vi "dC(T)_2024.vi"(2 "Temperature (K)":dbl=373.15 format="%.4g") -> (0 "dCa/dT":dbl=-9.989510208451924e-13 format="%#_4g", 1 "d^2Ca/dT^2":dbl=2.3734887970956986e-15 format="%#_4g", 3 "dCw/dT":dbl=1.21722616713758e-08 format="%_4g", 4 "d^2Cw/dT^2":dbl=-3.6083232318005423e-10 format="%_4g", 5 "T*dCa/dT":dbl=-3.7275857342838354e-10 format="%#_4g", 6 "T^2*d^2Ca/dT^2":dbl=3.3048676965102036e-10 format="%#_4g", 8 "T*dCw/dT":dbl=4.54207944267388e-06 format="%#_4g", 9 "T^2*d^2Cw/dT^2":dbl=-5.024262554740888e-05 format="%_4e")   [LabVIEW 2016]
uses:
  2022/SOS_Global_2022.vi
  <vilib>/Analysis/NI_AALPro.lvlib
  <vilib>/gmath/NI_Gmath.lvlib
panel:
  in  "C source ref water":i32(listbox)=1
  in  "C source ref dry air":i32(listbox)=1
  in  "method derivatives":u16(ring)=2 items=["2nd Order Central", "4th Order Central", "Forward", "Backward"]
  in  "interpolation method":i32(ring)=2 items=["nearest", "linear", "spline", "cubic Hermite", "Lagrange"]
  in  "method interpolation":i32(ring)=2 items=["nearest", "linear", "spline", "cubic Hermite", "Lagrange"]
  in  "method derivatives":u16(ring)=2 items=["2nd Order Central", "4th Order Central", "Forward", "Backward"]
  # "m^6/mol^2"
  # "m^6/(mol^2 K)"
  # "m^6/(mol^2 K^2)"
  # "m^6/mol^2"
  # "m^6/mol^2"
  # "m^6/(mol^2 K)"
  # "m^6/(mol^2 K^2)"
  # "m^6/mol^2"
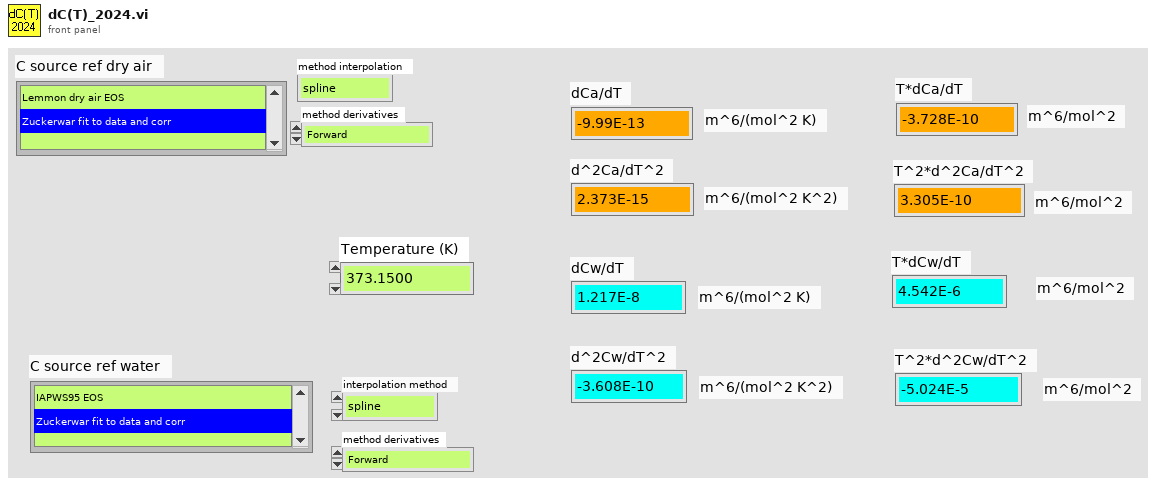
[diagram p1: front panel]
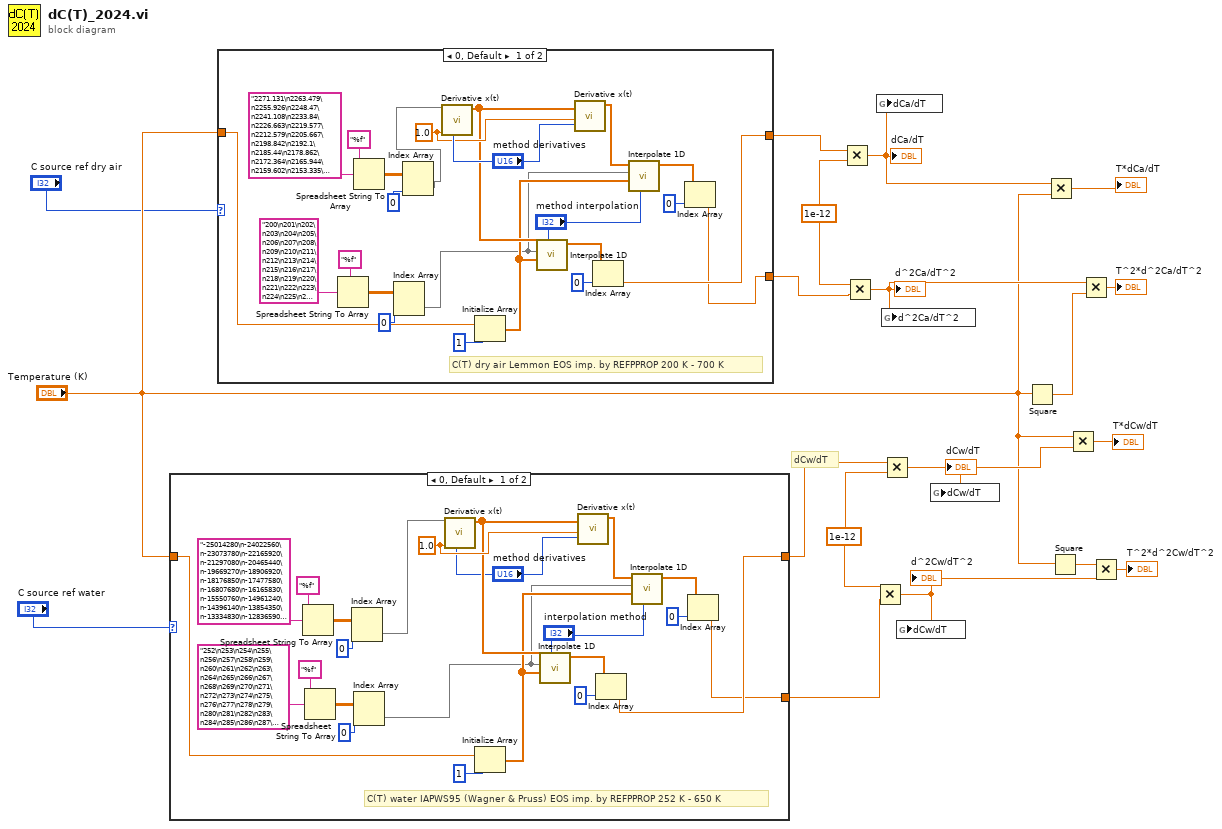
[diagram p0: block diagram]
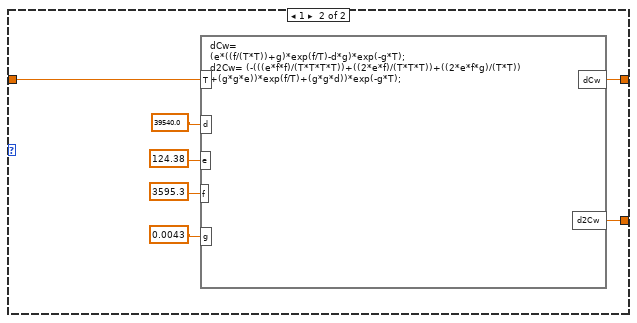
[diagram p2: hidden frame]
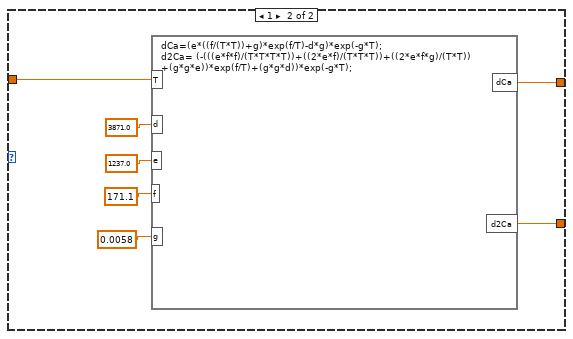
[diagram p3: hidden frame]
diagram:
  w14 = 1e-12 ("y")
  w16 = 1e-12 ("y")
  # "dCw/dT"
  n1 = case shown="0, Default" "C source ref water" {
    tunnel: [w32 w46] -> w18
    tunnel: [w31 w45] -> w15
    tunnel: "Temperature (K)" -> [w22 w44]
    frame 0, Default {
      w43 = 1.0 ("dt")
      # "C(T) water IAPWS95 (Wagner & Pruss) EOS imp. by REFPPROP 252 K - 650 K"
      n2 = Spreadsheet String To Array(format string="%f", spreadsheet string="-25014280\n-24022560\n-23073780\n-22165920\n-21297080\n-20465440\n-19669270\n-18906920\n-18176850\n-17477580\n-16807680\n-16165830\n-15550760\n-14961240\n-14396140\n-13854350\n-13334830\n-12836590\n-12358690\n-11900220\n-11460330\n-11038200\n-10633050\n-10244150\n-9870788\n-9512288\n-9168011\n-8837345\n-8519707\n-8214540\n-7921313\n-7639520\n-7368677\n-7108323\n-6858018\n-6617340\n-6385889\n-6163280\n-5949148\n-5743143\n-5544930\n-5354189\n-5170616\n-4993917\n-4823814\n-4660040\n-4502339\n-4350468\n-4204192\n-4063288\n-3927542\n-3796750\n-3670714\n-3549248\n-3432172\n-3319314\n-3210509\n-3105600\n-3004434\n-2906867\n-2812760\n-2721981\n-2634401\n-2549898\n-2468355\n-2389659\n-2313704\n-2240384\n-2169601\n-2101260\n-2035270\n-1971542\n-1909993\n-1850541\n-1793110\n-1737624\n-1684013\n-1632207\n-1582141\n-1533751\n-1486977\n-1441759\n-1398042\n-1355772\n-1314896\n-1275366\n-1237132\n-1200148\n-1164371\n-1129758\n-1096267\n-1063859\n-1032497\n-1002143\n-972761.7\n-944320.3\n-916785.9\n-890126.9\n-864313.3\n-839315.9\n-815106.7\n-791658.9\n-768946.4\n-746944.1\n-725628.1\n-704975.1\n-684962.7\n-665569.4\n-646774.4\n-628557.7\n-610899.9\n-593782.5\n-577187.6\n-561097.8\n-545496.5\n-530367.5\n-515695.4\n-501465.2\n-487662.5\n-474273.3\n-461284.2\n-448682.3\n-436454.9\n-424590.1\n-413076.2\n-401902\n-391056.4\n-380529.2\n-370310.1\n-360389.4\n-350757.6\n-341405.5\n-332324.5\n-323505.9\n-314941.6\n-306623.5\n-298544.1\n-290695.8\n-283071.6\n-275664.5\n-268467.7\n-261474.9\n-254679.6\n-248076\n-241658.1\n-235420.3\n-229357\n-223463.1\n-217733.3\n-212162.7\n-206746.6\n-201480.2\n-196359.1\n-191379\n-186535.6\n-181824.9\n-177242.9\n-172785.9\n-168450\n-164231.9\n-160127.9\n-156134.8\n-152249.3\n-148468.2\n-144788.6\n-141207.5\n-137722\n-134329.3\n-131026.8\n-127811.9\n-124682.1\n-121634.9\n-118667.9\n-115779\n-112965.8\n-110226.2\n-107558.1\n-104959.6\n-102428.6\n-99963.2\n-97561.63\n-95222.08\n-92942.8\n-90722.13\n-88558.43\n-86450.12\n-84395.67\n-82393.59\n-80442.43\n-78540.79\n-76687.32\n-74880.7\n-73119.64\n-71402.91\n-69729.29\n-68097.63\n-66506.77\n-64955.62\n-63443.11\n-61968.2\n-60529.87\n-59127.16\n-57759.1\n-56424.77\n-55123.27\n-53853.73\n-52615.31\n-51407.18\n-50228.54\n-49078.61\n-47956.64\n-46861.9\n-45793.68\n-44751.27\n-43734.01\n-42741.25\n-41772.34\n-40826.67\n-39903.64\n-39002.67\n-38123.18\n-37264.63\n-36426.48\n-35608.2\n-34809.29\n-34029.26\n-33267.62\n-32523.91\n-31797.67\n-31088.47\n-30395.87\n-29719.46\n-29058.82\n-28413.56\n-27783.31\n-27167.67\n-26566.3\n-25978.82\n-25404.91\n-24844.21\n-24296.42\n-23761.2\n-23238.24\n-22727.25\n-22227.94\n-21740\n-21263.18\n-20797.19\n-20341.78\n-19896.68\n-19461.64\n-19036.43\n-18620.8\n-18214.52\n-17817.37\n-17429.12\n-17049.58\n-16678.51\n-16315.73\n-15961.04\n-15614.24\n-15275.15\n-14943.57\n-14619.35\n-14302.29\n-13992.23\n-13689.01\n-13392.47\n-13102.45\n-12818.79\n-12541.35\n-12269.98\n-12004.54\n-11744.9\n-11490.92\n-11242.46\n-10999.4\n-10761.62\n-10528.99\n-10301.39\n-10078.71\n-9860.841\n-9647.665\n-9439.078\n-9234.975\n-9035.254\n-8839.814\n-8648.56\n-8461.395\n-8278.228\n-8098.968\n-7923.527\n-7751.819\n-7583.761\n-7419.269\n-7258.265\n-7100.67\n-6946.408\n-6795.406\n-6647.589\n-6502.888\n-6361.234\n-6222.559\n-6086.797\n-5953.883\n-5823.756\n-5696.353\n-5571.615\n-5449.483\n-5329.901\n-5212.812\n-5098.162\n-4985.898\n-4875.968\n-4768.322\n-4662.909\n-4559.681\n-4458.591\n-4359.593\n-4262.641\n-4167.693\n-4074.703\n-3983.631\n-3894.436\n-3807.076\n-3721.514\n-3637.71\n-3555.627\n-3475.228\n-3396.478\n-3319.342\n-3243.785\n-3169.773\n-3097.276\n-3026.259\n-2956.693\n-2888.546\n-2821.789\n-2756.392\n-2692.328\n-2629.568\n-2568.084\n-2507.851\n-2448.842\n-2391.032\n-2334.395\n-2278.908\n-2224.547\n-2171.288\n-2119.108\n-2067.985\n-2017.898\n-1968.824\n-1920.744\n-1873.636\n-1827.481\n-1782.26\n-1737.952\n-1694.54\n-1652.005\n-1610.329\n-1569.495\n-1529.485\n-1490.283\n-1451.873\n-1414.238\n-1377.362\n-1341.231\n-1305.829\n-1271.142\n-1237.154\n-1203.853\n-1171.223\n-1139.253\n-1107.928\n-1077.235\n-1047.162\n-1017.696\n-988.8261\n-960.5393\n-932.8241\n-905.6693\n-879.0637\n-852.9963\n-827.4564\n-802.4337\n-777.9178\n-753.8986\n-730.3665\n-707.3116\n-684.7246\n-662.5963\n-640.9176\n-619.6796\n-598.8737\n-578.4913\n-558.5243\n-538.9643\n-519.8034") -> (array=w26:dbl[][])  [unwired: 2 in]
      n3 = Spreadsheet String To Array(format string="%f", spreadsheet string="252\n253\n254\n255\n256\n257\n258\n259\n260\n261\n262\n263\n264\n265\n266\n267\n268\n269\n270\n271\n272\n273\n274\n275\n276\n277\n278\n279\n280\n281\n282\n283\n284\n285\n286\n287\n288\n289\n290\n291\n292\n293\n294\n295\n296\n297\n298\n299\n300\n301\n302\n303\n304\n305\n306\n307\n308\n309\n310\n311\n312\n313\n314\n315\n316\n317\n318\n319\n320\n321\n322\n323\n324\n325\n326\n327\n328\n329\n330\n331\n332\n333\n334\n335\n336\n337\n338\n339\n340\n341\n342\n343\n344\n345\n346\n347\n348\n349\n350\n351\n352\n353\n354\n355\n356\n357\n358\n359\n360\n361\n362\n363\n364\n365\n366\n367\n368\n369\n370\n371\n372\n373\n374\n375\n376\n377\n378\n379\n380\n381\n382\n383\n384\n385\n386\n387\n388\n389\n390\n391\n392\n393\n394\n395\n396\n397\n398\n399\n400\n401\n...") -> (array=w29:dbl[][])  [unwired: 2 in]
      n4 = Index Array(array=w26, index (col)=0 ("disabled index (col)")) -> (element=w20:dbl[])  [unwired: 1 in]
      n5 = Index Array(array=w29, index (col)=0 ("disabled index (col)")) -> (element=w21:dbl[])  [unwired: 1 in]
      n6 = call <vilib>:"Derivative x(t).vi"("method"="method derivatives", "dt"=w43, "X"=w20) -> ("dX/dt"=w36:dbl[])  [unwired: 7 in, 1 out]
      n7 = Initialize Array(w22, 1 ("dimension size")) -> (w35:dbl[])
      n8 = call <vilib>:"Interpolate 1D.vi"("method"="interpolation method", "xi"=w35, "X"=w21, "Y"=w36) -> ("yi"=w41:dbl[])  [unwired: 5 in, 2 out]
      n9 = call <vilib>:"Derivative x(t).vi"("method"="method derivatives", "dt"=w43, "X"=w36) -> ("dX/dt"=w37:dbl[])  [unwired: 7 in, 1 out]
      n10 = Index Array(array=w41, index=0) -> (element=w32:dbl)
      n11 = call <vilib>:"Interpolate 1D.vi"("method"="interpolation method", "xi"=w35, "X"=w21, "Y"=w37) -> ("yi"=w39:dbl[])  [unwired: 5 in, 2 out]
      n12 = Index Array(array=w39, index=0) -> (element=w31:dbl)
    }
    frame 1 {
      n13 = formula code="dCw= \n(e*((f/(T*T))+g)*exp(f/T)-d*g)*exp(-g*T);\nd2Cw= (-(((e*f*f)/(T*T*T*T))+((2*e*f)/(T*T*T))+((2*e*f*g)/(T*T))\n+(g*g*e))*exp(f/T)+(g*g*d))*exp(-g*T);"("T"=w44, "d"=39540.0 ("input variable"), "e"=124.38 ("input variable"), "f"=3595.3 ("input variable"), "g"=0.0043 ("input variable")) -> ("dCw"=w46:dbl, "d2Cw"=w45:dbl)
    }
  }
  n14 = case shown="0, Default" "C source ref dry air" {
    tunnel: [w63 w77] -> w19
    tunnel: [w62 w76] -> w17
    tunnel: "Temperature (K)" -> [w56 w75]
    frame 0, Default {
      w73 = 1.0 ("dt")
      # "C(T) dry air Lemmon EOS imp. by REFPPROP 200 K - 700 K"
      n15 = Spreadsheet String To Array(format string="%f", spreadsheet string="200\n201\n202\n203\n204\n205\n206\n207\n208\n209\n210\n211\n212\n213\n214\n215\n216\n217\n218\n219\n220\n221\n222\n223\n224\n225\n226\n227\n228\n229\n230\n231\n232\n233\n234\n235\n236\n237\n238\n239\n240\n241\n242\n243\n244\n245\n246\n247\n248\n249\n250\n251\n252\n253\n254\n255\n256\n257\n258\n259\n260\n261\n262\n263\n264\n265\n266\n267\n268\n269\n270\n271\n272\n273\n274\n275\n276\n277\n278\n279\n280\n281\n282\n283\n284\n285\n286\n287\n288\n289\n290\n291\n292\n293\n294\n295\n296\n297\n298\n299\n300\n301\n302\n303\n304\n305\n306\n307\n308\n309\n310\n311\n312\n313\n314\n315\n316\n317\n318\n319\n320\n321\n322\n323\n324\n325\n326\n327\n328\n329\n330\n331\n332\n333\n334\n335\n336\n337\n338\n339\n340\n341\n342\n343\n344\n345\n346\n347\n348\n349\n...") -> (array=w59:dbl[][])  [unwired: 2 in]
      n16 = Spreadsheet String To Array(format string="%f", spreadsheet string="2271.131\n2263.479\n2255.926\n2248.47\n2241.108\n2233.84\n2226.663\n2219.577\n2212.579\n2205.667\n2198.842\n2192.1\n2185.44\n2178.862\n2172.364\n2165.944\n2159.602\n2153.335\n2147.143\n2141.024\n2134.977\n2129.002\n2123.096\n2117.26\n2111.49\n2105.788\n2100.151\n2094.578\n2089.069\n2083.623\n2078.237\n2072.913\n2067.648\n2062.441\n2057.293\n2052.201\n2047.165\n2042.185\n2037.259\n2032.386\n2027.566\n2022.798\n2018.082\n2013.415\n2008.798\n2004.231\n1999.711\n1995.239\n1990.814\n1986.435\n1982.101\n1977.812\n1973.568\n1969.367\n1965.209\n1961.093\n1957.019\n1952.986\n1948.994\n1945.042\n1941.129\n1937.255\n1933.42\n1929.622\n1925.862\n1922.139\n1918.452\n1914.801\n1911.185\n1907.605\n1904.058\n1900.546\n1897.067\n1893.621\n1890.208\n1886.828\n1883.479\n1880.161\n1876.874\n1873.618\n1870.392\n1867.196\n1864.03\n1860.892\n1857.784\n1854.703\n1851.651\n1848.626\n1845.628\n1842.657\n1839.713\n1836.796\n1833.904\n1831.038\n1828.197\n1825.381\n1822.59\n1819.823\n1817.08\n1814.362\n1811.666\n1808.994\n1806.345\n1803.719\n1801.115\n1798.533\n1795.974\n1793.436\n1790.919\n1788.423\n1785.949\n1783.495\n1781.061\n1778.648\n1776.254\n1773.881\n1771.527\n1769.192\n1766.876\n1764.579\n1762.301\n1760.041\n1757.799\n1755.576\n1753.37\n1751.182\n1749.011\n1746.858\n1744.721\n1742.602\n1740.499\n1738.413\n1736.343\n1734.289\n1732.251\n1730.229\n1728.222\n1726.231\n1724.255\n1722.295\n1720.349\n1718.419\n1716.503\n1714.601\n1712.714\n1710.841\n1708.982\n1707.137\n1705.305\n1703.488\n1701.684\n1699.893\n1698.115\n1696.351\n1694.599\n1692.861\n1691.135\n1689.421\n1687.72\n1686.031\n1684.355\n1682.69\n1681.038\n1679.397\n1677.768\n1676.151\n1674.545\n1672.95\n1671.367\n1669.795\n1668.234\n1666.684\n1665.144\n1663.616\n1662.098\n1660.59\n1659.093\n1657.606\n1656.13\n1654.663\n1653.207\n1651.76\n1650.324\n1648.897\n1647.48\n1646.072\n1644.674\n1643.285\n1641.905\n1640.535\n1639.174\n1637.822\n1636.479\n1635.144\n1633.819\n1632.502\n1631.194\n1629.894\n1628.603\n1627.321\n1626.046\n1624.78\n1623.522\n1622.273\n1621.031\n1619.797\n1618.571\n1617.353\n1616.143\n1614.94\n1613.745\n1612.558\n1611.378\n1610.205\n1609.04\n1607.882\n1606.731\n1605.588\n1604.452\n1603.322\n1602.2\n1601.084\n1599.976\n1598.874\n1597.779\n1596.691\n1595.609\n1594.534\n1593.466\n1592.403\n1591.348\n1590.298\n1589.255\n1588.219\n1587.188\n1586.164\n1585.146\n1584.133\n1583.127\n1582.127\n1581.133\n1580.144\n1579.161\n1578.184\n1577.213\n1576.248\n1575.288\n1574.334\n1573.385\n1572.441\n1571.504\n1570.571\n1569.644\n1568.722\n1567.806\n1566.895\n1565.988\n1565.088\n1564.192\n1563.301\n1562.415\n1561.535\n1560.659\n1559.788\n1558.922\n1558.061\n1557.205\n1556.353\n1555.506\n1554.664\n1553.827\n1552.994\n1552.165\n1551.342\n1550.522\n1549.708\n1548.897\n1548.092\n1547.29\n1546.493\n1545.7\n1544.912\n1544.127\n1543.347\n1542.571\n1541.8\n1541.032\n1540.268\n1539.509\n1538.754\n1538.002\n1537.255\n1536.511\n1535.772\n1535.036\n1534.304\n1533.576\n1532.852\n1532.132\n1531.415\n1530.702\n1529.993\n1529.287\n1528.585\n1527.887\n1527.192\n1526.501\n1525.814\n1525.13\n1524.449\n1523.772\n1523.098\n1522.428\n1521.761\n1521.098\n1520.438\n1519.781\n1519.127\n1518.477\n1517.83\n1517.186\n1516.546\n1515.909\n1515.274\n1514.643\n1514.015\n1513.391\n1512.769\n1512.15\n1511.535\n1510.922\n1510.312\n1509.706\n1509.102\n1508.501\n1507.904\n1507.309\n1506.717\n1506.127\n1505.541\n1504.958\n1504.377\n1503.799\n1503.224\n1502.651\n1502.082\n1501.515\n1500.95\n1500.389\n1499.83\n1499.274\n1498.72\n1498.169\n1497.62\n1497.074\n1496.531\n1495.99\n1495.452\n1494.916\n1494.383\n1493.852\n1493.324\n1492.798\n1492.274\n1491.753\n1491.235\n1490.718\n1490.204\n1489.693\n1489.183\n1488.677\n1488.172\n1487.67\n1487.17\n1486.672\n1486.176\n1485.683\n1485.192\n1484.703\n1484.216\n1483.732\n1483.249\n1482.769\n1482.291\n1481.815\n1481.342\n1480.87\n1480.4\n1479.933\n1479.467\n1479.004\n1478.542\n1478.083\n1477.626\n1477.17\n1476.717\n1476.266\n1475.816\n1475.369\n1474.923\n1474.48\n1474.038\n1473.598\n1473.16\n1472.724\n1472.29\n1471.858\n1471.428\n1470.999\n1470.572\n1470.147\n1469.724\n1469.303\n1468.884\n1468.466\n1468.05\n1467.636\n1467.223\n1466.812\n1466.403\n1465.996\n1465.59\n1465.186\n1464.784\n1464.384\n1463.985\n1463.588\n1463.192\n1462.798\n1462.406\n1462.015\n1461.626\n1461.238\n1460.853\n1460.468\n1460.086\n1459.704\n1459.325\n1458.947\n1458.57\n1458.195\n1457.822\n1457.45\n1457.079\n1456.71\n1456.343\n1455.977\n1455.612\n1455.249\n1454.887\n1454.527\n1454.168\n1453.811\n1453.455\n1453.101\n1452.748\n1452.396\n1452.046\n1451.697\n1451.349\n1451.003\n1450.658\n1450.315\n1449.973\n1449.632\n1449.293\n1448.955\n1448.618\n1448.282\n1447.948\n1447.615\n1447.284\n1446.953\n1446.624\n1446.297\n1445.97\n1445.645\n1445.321\n1444.998\n1444.677\n1444.356\n1444.037\n1443.719\n1443.403\n1443.087\n1442.773\n1442.46\n1442.148\n1441.837\n1441.528\n1441.22\n1440.912\n1440.606\n1440.302\n1439.998\n1439.695\n1439.394\n1439.093\n1438.794\n1438.496\n1438.199") -> (array=w54:dbl[][])  [unwired: 2 in]
      n17 = Index Array(array=w59, index (col)=0 ("disabled index (col)")) -> (element=w57:dbl[])  [unwired: 1 in]
      n18 = Index Array(array=w54, index (col)=0 ("disabled index (col)")) -> (element=w52:dbl[])  [unwired: 1 in]
      n19 = call <vilib>:"Derivative x(t).vi"("method"="method derivatives", "dt"=w73, "X"=w52) -> ("dX/dt"=w66:dbl[])  [unwired: 7 in, 1 out]
      n20 = Initialize Array(w56, 1 ("dimension size")) -> (w65:dbl[])
      n21 = call <vilib>:"Interpolate 1D.vi"("method"="method interpolation", "xi"=w65, "X"=w57, "Y"=w66) -> ("yi"=w71:dbl[])  [unwired: 5 in, 2 out]
      n22 = call <vilib>:"Derivative x(t).vi"("method"="method derivatives", "dt"=w73, "X"=w66) -> ("dX/dt"=w67:dbl[])  [unwired: 7 in, 1 out]
      n23 = Index Array(array=w71, index=0) -> (element=w63:dbl)
      n24 = call <vilib>:"Interpolate 1D.vi"("method"="method interpolation", "xi"=w65, "X"=w57, "Y"=w67) -> ("yi"=w69:dbl[])  [unwired: 5 in, 2 out]
      n25 = Index Array(array=w69, index=0) -> (element=w62:dbl)
    }
    frame 1 {
      n26 = formula code="dCa=(e*((f/(T*T))+g)*exp(f/T)-d*g)*exp(-g*T);\nd2Ca= (-(((e*f*f)/(T*T*T*T))+((2*e*f)/(T*T*T))+((2*e*f*g)/(T*T))\n+(g*g*e))*exp(f/T)+(g*g*d))*exp(-g*T);"("T"=w75, "d"=3871.0 ("input variable"), "e"=1237.0 ("input variable"), "f"=171.1 ("input variable"), "g"=0.0058 ("input variable")) -> ("dCa"=w77:dbl, "d2Ca"=w76:dbl)
    }
  }
  n27 = Multiply(x=w19, y=w16) -> (x*y=w13:dbl)
  "dCa/dT" <- w13
  n28 = Multiply(x=w16, y=w17) -> (x*y=w10:dbl)
  "d^2Ca/dT^2" <- w10
  n29 = Multiply(x=w14, y=w15) -> (x*y=w5:dbl)
  "d^2Cw/dT^2" <- w5
  n30 = global write "SOS_Global_2022.vi" "dCa/dT"(w13) -> ()
  n31 = global write "SOS_Global_2022.vi" "d^2Ca/dT^2"(w10) -> ()
  n32 = Multiply(x=w18, y=w14) -> (x*y=w8:dbl)
  "dCw/dT" <- w8
  n33 = global write "SOS_Global_2022.vi" "dCw/dT"(w5) -> ()
  n34 = global write "SOS_Global_2022.vi" "dCw/dT"(w8) -> ()
  n35 = Square(x="Temperature (K)") -> (x^2=w11:dbl)
  n36 = Multiply(x=w13, y="Temperature (K)") -> (x*y=→"T*dCa/dT":dbl)
  n37 = Square(x="Temperature (K)") -> (x^2=w4:dbl)
  n38 = Multiply(x="Temperature (K)", y=w8) -> (x*y=→"T*dCw/dT":dbl)
  n39 = Multiply(x=w10, y=w11) -> (x*y=→"T^2*d^2Ca/dT^2":dbl)
  n40 = Multiply(x=w4, y=w5) -> (x*y=→"T^2*d^2Cw/dT^2":dbl)
